vi "Open.vi"(8 "error in (no error)":errorcluster) -> (0 "error out":errorcluster)   [LabVIEW 2019, in "Kinova MICO² USB.lvlib"]
uses:
  <vilib>/Utility/error.llb/Error Cluster From Error Code.vi
  <vilib>/ErrorRing/Error Ring.xnode
  Kernel32.dll
  lib/ld-2.24.so
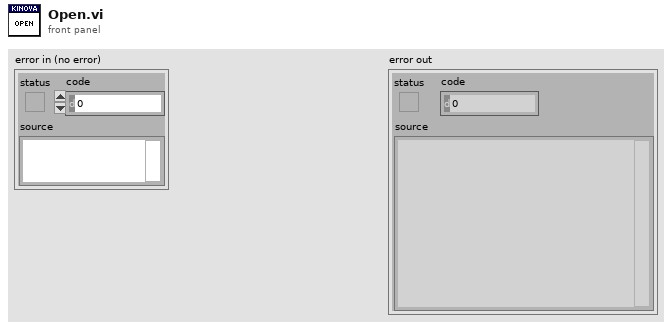
[diagram p1: front panel]
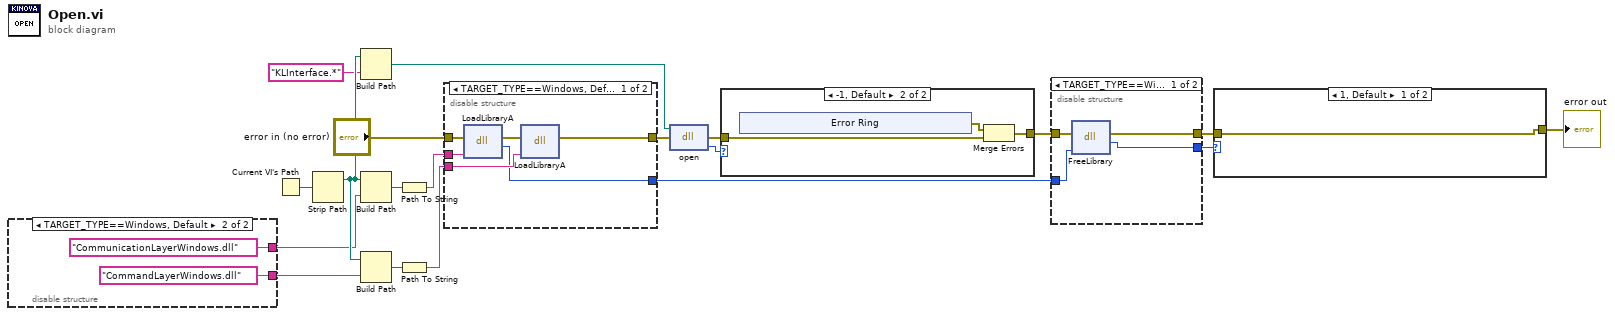
[diagram p0: block diagram]
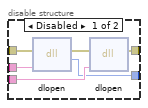
[diagram p3: hidden frame]
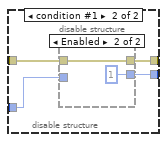
[diagram p4: hidden frame]
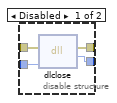
[diagram p5: hidden frame]
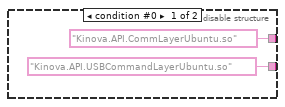
[diagram p6: hidden frame]
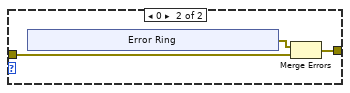
[diagram p7: hidden frame]
diagram:
  n1 = disable-structure shown="TARGET_TYPE==Windows, Default" {
    disable-tunnel: ["Kinova.API.USBCommandLayerUbuntu.so" ("name or relative path") "CommandLayerWindows.dll" ("name or relative path")] -> w8
    disable-tunnel: ["Kinova.API.CommLayerUbuntu.so" ("name or relative path") "CommunicationLayerWindows.dll" ("name or relative path")] -> w7
    frame condition #0 {
    }
    frame condition #1 (active) {
    }
  }
  n2 = Current VI's Path() -> (path=w15:path)
  n3 = Strip Path(path=w15) -> (stripped path=w10:path)  [unwired: 1 out]
  n4 = Build Path(base path=w10, name or relative path="KLInterface.*") -> (appended path=w1:path)
  n5 = Build Path(base path=w10, name or relative path=w7) -> (appended path=w18:path)
  n6 = Build Path(base path=w10, name or relative path=w8) -> (appended path=w11:path)
  n7 = Path To String(path=w18) -> (string=w3:string)
  n8 = Path To String(path=w11) -> (string=w9:string)
  n9 = disable-structure shown="TARGET_TYPE==Windows, Default" {
    disable-tunnel: w9 -> [w29 w34]
    disable-tunnel: [w28 w33] -> w5
    disable-tunnel: "error in (no error)" -> [w26 w32]
    disable-tunnel: w3 -> [w27 w31]
    disable-tunnel: [w24 w30] -> w2
    frame condition #0 (active) {
      n10 = dll-call lib="Kernel32.dll" fn="LoadLibraryA"(error in=w26, "file"=w27) -> (error out=w25:errorcluster, "return type"=w24:u32)  [unwired: 3 in, 1 out]
      n11 = dll-call lib="Kernel32.dll" fn="LoadLibraryA"(error in=w25, "file"=w29) -> (error out=w28:errorcluster)  [unwired: 4 in, 1 out]
    }
    frame condition #1 {
      n12 = disable-structure shown="Enabled" {
        disable-tunnel: w34 -> [w40 _]
        disable-tunnel: [w39 w41] -> w33
        disable-tunnel: w32 -> [w38 w41]
        disable-tunnel: w31 -> [w37 _]
        disable-tunnel: [w36 _] -> w30
        frame Disabled {
          n13 = dll-call lib="lib/ld-2.24.so" fn="dlopen"(error in=w38, "file"=w37) -> (error out=w35:errorcluster, "return type"=w36:u32)  [unwired: 3 in, 1 out]
          n14 = dll-call lib="lib/ld-2.24.so" fn="dlopen"(error in=w35, "file"=w40) -> (error out=w39:errorcluster)  [unwired: 4 in, 1 out]
        }
        frame Enabled {
        }
      }
    }
  }
  n15 = dll-call lib="C:/Users/mcjssdcc/source/repos/Kinova Labview Interface/Debug/KLInterface.dll" fn="open"(path in=w1, error in=w5) -> (error out=w17:errorcluster, "return type"=w16:i32)  [unwired: 1 in, 1 out]
  n16 = case shown="-1, Default" w16 {
    tunnel: [w42 w44] -> w19
    tunnel: w17 -> [w42 w43]
    frame 1 {
    }
    frame -1, Default {
      n17 = xnode "Error Ring"() -> ("error out"=w45:errorcluster)
      n18 = Merge Errors(w45, w43) -> (w44:errorcluster)
    }
  }
  n19 = disable-structure shown="TARGET_TYPE==Windows, Default" {
    disable-tunnel: w2 -> [w54 w58]
    disable-tunnel: w19 -> [w53 w57]
    disable-tunnel: [w52 w56] -> w13
    disable-tunnel: [w51 w55] -> w12
    frame condition #0 (active) {
      n20 = dll-call lib="Kernel32.dll" fn="FreeLibrary"(error in=w53, "hmodule"=w54) -> (error out=w51:errorcluster, "return type"=w52:i32)  [unwired: 3 in, 1 out]
    }
    frame condition #1 {
      n21 = disable-structure shown="Enabled" {
        disable-tunnel: w58 -> [w62 _]
        disable-tunnel: w57 -> [w61 w64]
        disable-tunnel: [w60 1 ("return type")] -> w56
        disable-tunnel: [w59 w64] -> w55
        frame Disabled {
          n22 = dll-call lib="lib/ld-2.24.so" fn="dlclose"(error in=w61, "hmodule"=w62) -> (error out=w59:errorcluster, "return type"=w60:i32)  [unwired: 3 in, 1 out]
        }
        frame Enabled {
        }
      }
    }
  }
  n23 = case shown="1, Default" w13 {
    tunnel: [w65 w67] -> w14
    tunnel: w12 -> [w65 w66]
    frame 1, Default {
    }
    frame 0 {
      n24 = xnode "Error Ring"() -> ("error out"=w68:errorcluster)
      n25 = Merge Errors(w68, w66) -> (w67:errorcluster)
    }
  }
  "error out" <- w14
